vi "frequency_sweep.vi"(0 "Frequency":dbl, 1 "Channel (1:Channel 1)":i32, 2 "Amplitude (1.0 Vpp)":dbl=1.0 min=0.001 max=20.0 step=1.0 format="%#.3f", 3 "DC Offset (0.00 V)":dbl min=-10.0 max=10.0, 4 "SG Device":T1(ring) caption="Signal Generator Device", 5 "Modulation frequency":dbl, 7 "Delay":dbl, 9 "Modulation Depth (0.0 %)":dbl, 11 "error in (no error)":errorcluster, 12 "Siglent Name":refnum<visa-resource-name>="USB0::0xF4EC::0x1102::SDG2XCAD4R3627::INSTR", 13 "AD2":i32, 14 "Stop 2":bool) -> (15 "error out":errorcluster)   [LabVIEW 2024, in "Sweep.lvlib"]
uses:
  Sweep.lvlib
  AD2/Node Parameters.ctl
  <instrlib>/Siglent SDG 1000 5000 800 Series/Public/Configure/Configure Modulation (AM).vi
  <instrlib>/Siglent SDG 1000 5000 800 Series/Siglent SDG 1000 5000 800 Series.lvlib
  AD2/AD2 DLL.lvlib
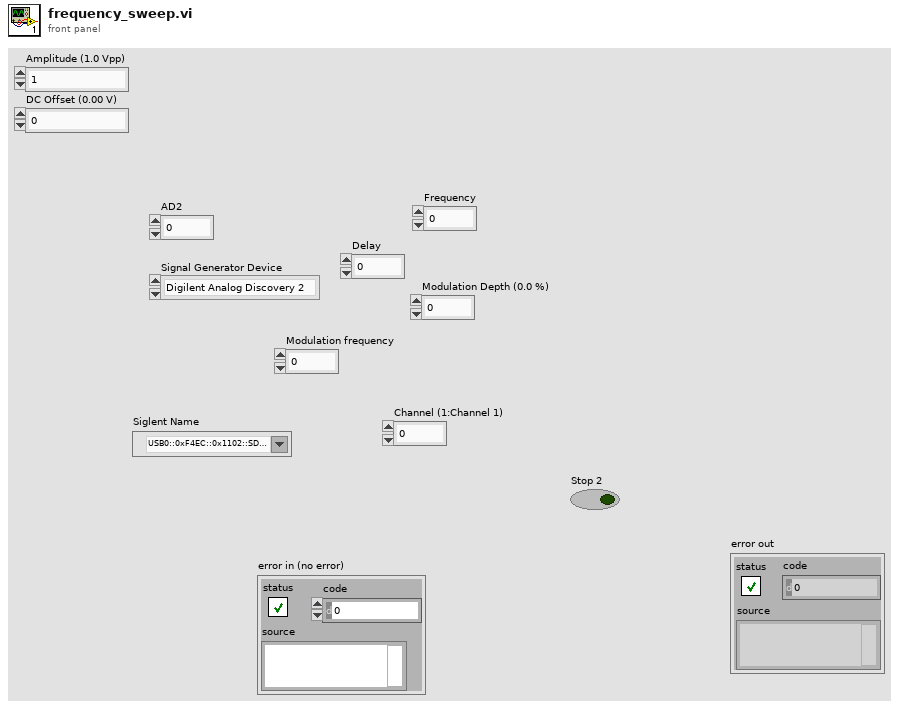
[diagram p1: front panel]
types:
  T1 = enum16{"Digilent Analog Discovery 2", "Siglent DG"}
  T2 = typedef "AD2 DLL.lvlib/Node Parameters.ctl" = cluster{"Function":u8, "Frequency":dbl, "Amplitude":dbl, "DC Offset":dbl, "Duty Cycle":dbl, "Phase":dbl}
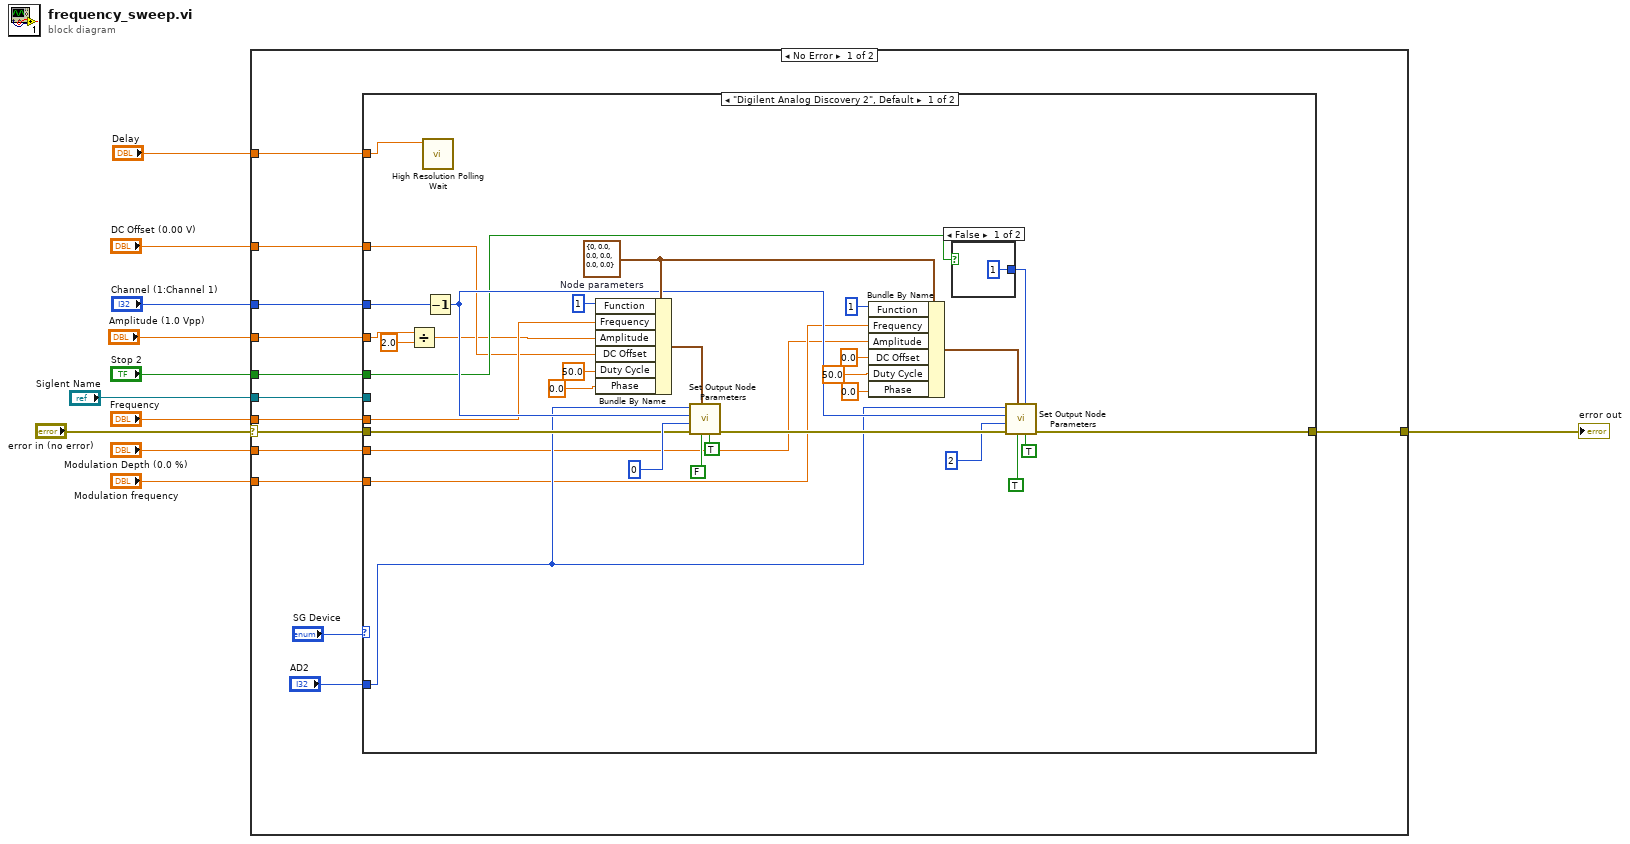
[diagram p0: block diagram]
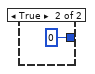
[diagram p2: hidden frame]
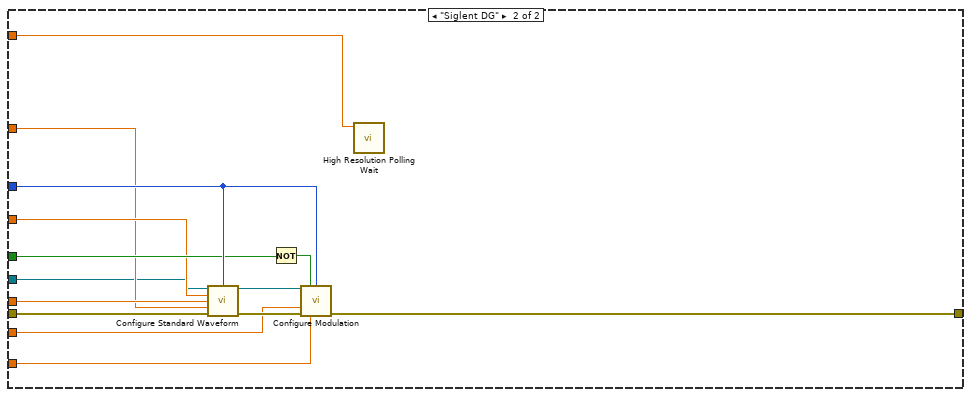
[diagram p3: hidden frame]
diagram:
  n1 = case shown="No Error" "error in (no error)" {
    selector: "error in (no error)" -> [w14 w73]
    tunnel: [w24 w73] -> w11
    tunnel: "Channel (1:Channel 1)" -> [w23 _]
    tunnel: "Modulation Depth (0.0 %)" -> [w22 _]
    tunnel: "Modulation frequency" -> [w21 _]
    tunnel: "Frequency" -> [w20 _]
    tunnel: "Stop 2" -> [w19 _]
    tunnel: "Amplitude (1.0 Vpp)" -> [w18 _]
    tunnel: "DC Offset (0.00 V)" -> [w17 _]
    tunnel: "Siglent Name" -> [w16 _]
    tunnel: "Delay" -> [w15 _]
    frame No Error {
      n2 = case shown="\"Digilent Analog Discovery 2\", Default" "SG Device" {
        tunnel: [w36 w71] -> w24
        tunnel: w23 -> [w28 w68]
        tunnel: w22 -> [w31 w67]
        tunnel: w21 -> [w32 w66]
        tunnel: w20 -> [w30 w65]
        tunnel: w19 -> [w34 w64]
        tunnel: w18 -> [w26 w63]
        tunnel: w17 -> [w29 w62]
        tunnel: w16 -> [_ w61]
        tunnel: w15 -> [w35 w60]
        tunnel: w14 -> [w37 w59]
        tunnel: "AD2" -> [w33 _]
        frame "Digilent Analog Discovery 2", Default {
          w45 = T2 {"Function"=0, "Frequency"=0.0, "Amplitude"=0.0, "DC Offset"=0.0, "Duty Cycle"=0.0, "Phase"=0.0}  # Node parameters
          n3 = Divide(x=w26, y=2.0) -> (x/y=w27:dbl)
          n4 = call <vilib>:"High Resolution Polling Wait.vi"("seconds to wait"=w35) -> ()  [unwired: 10 in, 1 out]
          n5 = Decrement(x=w28) -> (x-1=w42:i32)
          n6 = Bundle By Name(cluster=w45, "Function"=u8 1, "Frequency"=w30, "Amplitude"=w27, "DC Offset"=w29, "Duty Cycle"=50.0, "Phase"=0.0) -> (w53:T2)
          n7 = call "Set Output Node Parameters.vi"("Apply parameters"=TRUE, "Use Enable"=FALSE, "Node parameters"=w53, "error in (no error)"=w37, "node"=0, "idxChannel"=w42, "hdwf"=w33) -> ("error out"=w49:errorcluster)  [unwired: 3 in, 1 out]
          n8 = Bundle By Name(cluster=w45, "Function"=u8 1, "Frequency"=w32, "Amplitude"=w31, "DC Offset"=0.0, "Duty Cycle"=50.0, "Phase"=0.0) -> (w43:T2)
          n9 = case shown="False" w34 {
            tunnel: [1 ("Enable") 0 ("Enable")] -> w38
            frame False {
            }
            frame True {
            }
          }
          n10 = call "Set Output Node Parameters.vi"("Apply parameters"=TRUE, "Enable"=w38, "Use Enable"=TRUE, "Node parameters"=w43, "error in (no error)"=w49, "node"=2, "idxChannel"=w42, "hdwf"=w33) -> ("error out"=w36:errorcluster)  [unwired: 2 in, 1 out]
        }
        frame "Siglent DG" {
          n11 = call <instrlib>:"Configure Standard Waveform.vi"("VISA resource name"=w61, "Channel (1:Channel 1)"=w68, "Amplitude (1.0 Vpp)"=w63, "Frequency (1000 Hz)"=w65, "DC Offset (0.00 V)"=w62, "error in (no error)"=w59) -> ("VISA resource name out"=w69:refnum<visa-resource-name>, "error out"=w70:errorcluster)  [unwired: 8 in]
          n12 = Not(x=w64) -> (.not. x?=w72:bool)
          n13 = call-poly <instrlib>:"Configure Modulation.vi"("VISA resource name"=w69, "Enable Amplitude Modulation (T:Enable)"=w72, "Channel (1:Channel 1)"=w68, "Modulation Depth (0.0 %)"=w67, "error in (no error)"=w70, "Modulation Frequency (100 Hz)"=w66) -> ("error out"=w71:errorcluster)  [unwired: 8 in, 1 out]
          n14 = call <vilib>:"High Resolution Polling Wait.vi"("seconds to wait"=w60) -> ()  [unwired: 10 in, 1 out]
        }
      }
    }
    frame Error {
    }
  }
  "error out" <- w11
